vi "BCM_284_ctl.vi"(8 "error in":errorcluster caption="错误输入（无错误）", 9 "Input2":T2, 11 "Input1":T3) -> (0 "error out":errorcluster caption="错误输出", 1 "BCM284":T1 {"BCM电源模式" items=["关闭", "ACC", "开启", "预留", "START"]; "设防提示类型设置" items=["无", "亮灯并鸣笛", "亮灯", "鸣笛"]; "RLS下雨关窗模式" items=["关", "开", "预留", "错误"]; "防盗报警状态" items=["报警", "预报警", "禁止报警", "提醒", "警报", "部分报警", "未用"]; "自动开关窗设置" items=["禁止", "RKE长按控制", "车钥匙控制", "预留"]; "伴我回家时间选择" items=["无", "30s", "60s", "90s"]; "BCM提示引擎盖开关" items=["关闭", "半开", "预留", "无效"]; "后车窗加热器激活" items=["未激活", "激活", "预留", "无效"]}, 3 "CmdStr":string)   [LabVIEW 2013]
uses:
  Input1.ctl
  Input2.ctl
  BCM_284.ctl
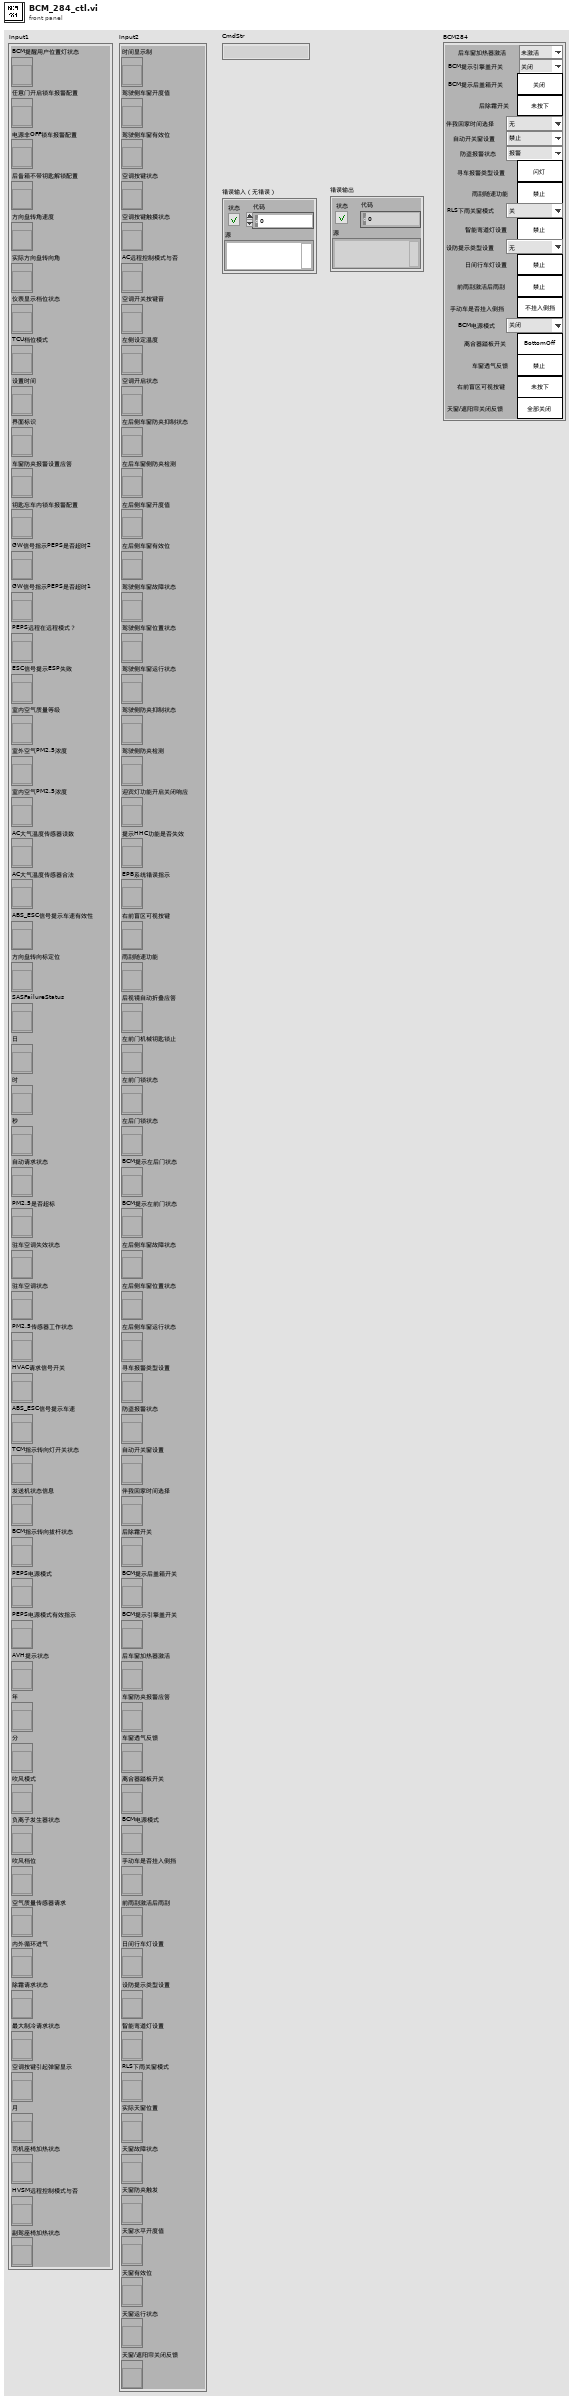
[diagram p1: front panel]
types:
  T1 = typedef "BCM_284.ctl" = cluster{"后车窗加热器激活":u16, "BCM提示引擎盖开关":u16, "BCM提示后盖箱开关":bool, "后除霜开关":bool, "伴我回家时间选择":u16, "自动开关窗设置":u16, "防盗报警状态":u16, "寻车报警类型设置":bool, "雨刮随速功能":bool, "RLS下雨关窗模式":u16, "智能弯道灯设置":bool, "设防提示类型设置":u16, "日间行车灯设置":bool, "前雨刮激活后雨刮":bool, "手动车是否挂入倒挡":bool, "BCM电源模式":u16, "离合器踏板开关":bool, "车窗透气反馈":bool, "右前盲区可视按键":bool, "天窗/遮阳帘关闭反馈":bool}
  T2 = typedef "Input2.ctl" = cluster{"时间显示制":refnum<vi>, "驾驶侧车窗开度值":refnum<vi>, "驾驶侧车窗有效位":refnum<vi>, "空调按键状态":refnum<vi>, "空调按键触摸状态":refnum<vi>, "AC远程控制模式与否":refnum<vi>, "空调开关按键音":refnum<vi>, "左侧设定温度":refnum<vi>, "空调开启状态":refnum<vi>, "左后侧车窗防夹抑制状态":refnum<vi>, "左后车窗侧防夹检测":refnum<vi>, "左后侧车窗开度值":refnum<vi>, "左后侧车窗有效位":refnum<vi>, "驾驶侧车窗故障状态":refnum<vi>, "驾驶侧车窗位置状态":refnum<vi>, "驾驶侧车窗运行状态":refnum<vi>, "驾驶侧防夹抑制状态":refnum<vi>, "驾驶侧防夹检测":refnum<vi>, "迎宾灯功能开启关闭响应":refnum<vi>, "提示HHC功能是否失效":refnum<vi>, "EPB系统错误指示":refnum<vi>, "右前盲区可视按键":refnum<vi>, "雨刮随速功能":refnum<vi>, "后视镜自动折叠应答":refnum<vi>, "左前门机械钥匙锁止":refnum<vi>, "左前门锁状态":refnum<vi>, "左后门锁状态":refnum<vi>, "BCM提示左后门状态":refnum<vi>, "BCM提示左前门状态":refnum<vi>, "左后侧车窗故障状态":refnum<vi>, "左后侧车窗位置状态":refnum<vi>, "左后侧车窗运行状态":refnum<vi>, "寻车报警类型设置":refnum<vi>, "防盗报警状态":refnum<vi>, "自动开关窗设置":refnum<vi>, "伴我回家时间选择":refnum<vi>, "后除霜开关":refnum<vi>, "BCM提示后盖箱开关":refnum<vi>, "BCM提示引擎盖开关":refnum<vi>, "后车窗加热器激活":refnum<vi>, "车窗防夹报警应答":refnum<vi>, "车窗透气反馈":refnum<vi>, "离合器踏板开关":refnum<vi>, "BCM电源模式":refnum<vi>, "手动车是否挂入倒挡":refnum<vi>, "前雨刮激活后雨刮":refnum<vi>, "日间行车灯设置":refnum<vi>, "设防提示类型设置":refnum<vi>, "智能弯道灯设置":refnum<vi>, "RLS下雨关窗模式":refnum<vi>, "实际天窗位置":refnum<vi>, "天窗故障状态":refnum<vi>, "天窗防夹触发":refnum<vi>, "天窗水平开度值":refnum<vi>, "天窗有效位":refnum<vi>, "天窗运行状态":refnum<vi>, "天窗/遮阳帘关闭反馈":refnum<vi>}
  T3 = typedef "Input1.ctl" = cluster{"BCM提醒用户位置灯状态":refnum<vi>, "任意门开启锁车报警配置":refnum<vi>, "电源非OFF锁车报警配置":refnum<vi>, "后备箱不带钥匙解锁配置":refnum<vi>, "方向盘转角速度":refnum<vi>, "实际方向盘转向角":refnum<vi>, "仪表显示档位状态":refnum<vi>, "TCU档位模式":refnum<vi>, "设置时间":refnum<vi>, "界面标识":refnum<vi>, "车窗防夹报警设置应答":refnum<vi>, "钥匙忘车内锁车报警配置":refnum<vi>, "GW信号指示PEPS是否超时2":refnum<vi>, "GW信号指示PEPS是否超时1":refnum<vi>, "PEPS远程在远程模式？":refnum<vi>, "ESC信号提示ESP失败":refnum<vi>, "室内空气质量等级":refnum<vi>, "室外空气PM2.5浓度":refnum<vi>, "室内空气PM2.5浓度":refnum<vi>, "AC大气温度传感器读数":refnum<vi>, "AC大气温度传感器合法":refnum<vi>, "ABS_ESC信号提示车速有效性":refnum<vi>, "方向盘转向标定位":refnum<vi>, "SASFailureStatus":refnum<vi>, "日":refnum<vi>, "时":refnum<vi>, "秒":refnum<vi>, "自动请求状态":refnum<vi>, "PM2.5是否超标":refnum<vi>, "驻车空调失效状态":refnum<vi>, "驻车空调状态":refnum<vi>, "PM2.5传感器工作状态":refnum<vi>, "HVAC请求信号开关":refnum<vi>, "ABS_ESC信号提示车速":refnum<vi>, "TCM指示转向灯开关状态":refnum<vi>, "发送机状态信息":refnum<vi>, "BCM指示转向拔杆状态":refnum<vi>, "PEPS电源模式":refnum<vi>, "PEPS电源模式有效指示":refnum<vi>, "AVH提示状态":refnum<vi>, "年":refnum<vi>, "分":refnum<vi>, "吹风模式":refnum<vi>, "负离子发生器状态":refnum<vi>, "吹风档位":refnum<vi>, "空气质量传感器请求":refnum<vi>, "内外循环进气":refnum<vi>, "除霜请求状态":refnum<vi>, "最大制冷请求状态":refnum<vi>, "空调按键引起弹窗显示":refnum<vi>, "月":refnum<vi>, "司机座椅加热状态":refnum<vi>, "HVSM远程控制模式与否":refnum<vi>, "副驾座椅加热状态":refnum<vi>}
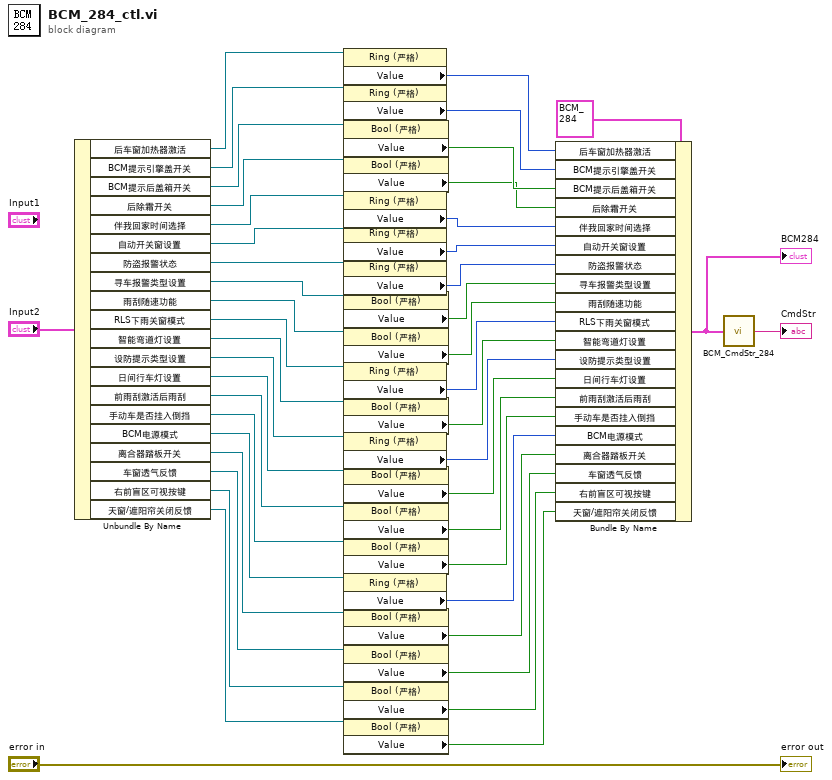
[diagram p0: block diagram]
diagram:
  n1 = Unbundle By Name("Input2") -> ("后车窗加热器激活"=w43:refnum<vi>, "BCM提示引擎盖开关"=w41:refnum<vi>, "BCM提示后盖箱开关"=w39:refnum<vi>, "后除霜开关"=w37:refnum<vi>, "伴我回家时间选择"=w35:refnum<vi>, "自动开关窗设置"=w33:refnum<vi>, "防盗报警状态"=w31:refnum<vi>, "寻车报警类型设置"=w29:refnum<vi>, "雨刮随速功能"=w27:refnum<vi>, "RLS下雨关窗模式"=w25:refnum<vi>, "智能弯道灯设置"=w23:refnum<vi>, "设防提示类型设置"=w21:refnum<vi>, "日间行车灯设置"=w19:refnum<vi>, "前雨刮激活后雨刮"=w17:refnum<vi>, "手动车是否挂入倒挡"=w15:refnum<vi>, "BCM电源模式"=w13:refnum<vi>, "离合器踏板开关"=w11:refnum<vi>, "车窗透气反馈"=w9:refnum<vi>, "右前盲区可视按键"=w7:refnum<vi>, "天窗/遮阳帘关闭反馈"=w5:refnum<vi>)
  n2 = property class="Ring (严格)"(reference=w43) -> ("Value"=w42:u16)  [unwired: 1 in, 2 out]
  n3 = property class="Ring (严格)"(reference=w41) -> ("Value"=w40:u16)  [unwired: 1 in, 2 out]
  n4 = property class="Bool (严格)"(reference=w39) -> ("Value"=w38:bool)  [unwired: 1 in, 2 out]
  n5 = property class="Bool (严格)"(reference=w37) -> ("Value"=w36:bool)  [unwired: 1 in, 2 out]
  n6 = property class="Ring (严格)"(reference=w35) -> ("Value"=w34:u16)  [unwired: 1 in, 2 out]
  n7 = property class="Ring (严格)"(reference=w33) -> ("Value"=w32:u16)  [unwired: 1 in, 2 out]
  n8 = property class="Ring (严格)"(reference=w31) -> ("Value"=w30:u16)  [unwired: 1 in, 2 out]
  n9 = property class="Bool (严格)"(reference=w29) -> ("Value"=w28:bool)  [unwired: 1 in, 2 out]
  n10 = property class="Bool (严格)"(reference=w27) -> ("Value"=w26:bool)  [unwired: 1 in, 2 out]
  n11 = property class="Ring (严格)"(reference=w25) -> ("Value"=w24:u16)  [unwired: 1 in, 2 out]
  n12 = property class="Bool (严格)"(reference=w23) -> ("Value"=w22:bool)  [unwired: 1 in, 2 out]
  n13 = property class="Ring (严格)"(reference=w21) -> ("Value"=w20:u16)  [unwired: 1 in, 2 out]
  n14 = property class="Bool (严格)"(reference=w19) -> ("Value"=w18:bool)  [unwired: 1 in, 2 out]
  n15 = property class="Bool (严格)"(reference=w17) -> ("Value"=w16:bool)  [unwired: 1 in, 2 out]
  n16 = property class="Bool (严格)"(reference=w15) -> ("Value"=w14:bool)  [unwired: 1 in, 2 out]
  n17 = property class="Ring (严格)"(reference=w13) -> ("Value"=w12:u16)  [unwired: 1 in, 2 out]
  n18 = property class="Bool (严格)"(reference=w11) -> ("Value"=w10:bool)  [unwired: 1 in, 2 out]
  n19 = property class="Bool (严格)"(reference=w9) -> ("Value"=w8:bool)  [unwired: 1 in, 2 out]
  n20 = property class="Bool (严格)"(reference=w7) -> ("Value"=w6:bool)  [unwired: 1 in, 2 out]
  n21 = property class="Bool (严格)"(reference=w5) -> ("Value"=w4:bool)  [unwired: 1 in, 2 out]
  n22 = Bundle By Name(cluster=T1 {"后车窗加热器激活"=0, "BCM提示引擎盖开关"=0, "BCM提示后盖箱开关"=FALSE, "后除霜开关"=FALSE, "伴我回家时间选择"=0, "自动开关窗设置"=0, "防盗报警状态"=0, "寻车报警类型设置"=FALSE, "雨刮随速功能"=FALSE, "RLS下雨关窗模式"=0, "智能弯道灯设置"=FALSE, "设防提示类型设置"=0, "日间行车灯设置"=FALSE, "前雨刮激活后雨刮"=FALSE, "手动车是否挂入倒挡"=FALSE, "BCM电源模式"=0, "离合器踏板开关"=FALSE, "车窗透气反馈"=FALSE, "右前盲区可视按键"=FALSE, "天窗/遮阳帘关闭反馈"=FALSE} ("BCM命令输入"), "后车窗加热器激活"=w42, "BCM提示引擎盖开关"=w40, "BCM提示后盖箱开关"=w38, "后除霜开关"=w36, "伴我回家时间选择"=w34, "自动开关窗设置"=w32, "防盗报警状态"=w30, "寻车报警类型设置"=w28, "雨刮随速功能"=w26, "RLS下雨关窗模式"=w24, "智能弯道灯设置"=w22, "设防提示类型设置"=w20, "日间行车灯设置"=w18, "前雨刮激活后雨刮"=w16, "手动车是否挂入倒挡"=w14, "BCM电源模式"=w12, "离合器踏板开关"=w10, "车窗透气反馈"=w8, "右前盲区可视按键"=w6, "天窗/遮阳帘关闭反馈"=w4) -> (w3:T1)
  "BCM284" <- w3
  n23 = call "BCM_CmdStr_284.vi"("BCM命令输入"=w3) -> ("CmdStr"=→"CmdStr":string)
  "error out" <- "error in"
